vi "LP Send Cmd Done.vi"(8 "error in (no error)":errorcluster, 10 "CMD":string, 11 "Data":variant) -> ()   [LabVIEW 2015]
uses:
  Stream/Controls/RT Streamer Queue element.ctl
  Stream/Controls/RT Streamer State.ctl
  Stream/RT Controls/RT Streamer Ack element.ctl
  Stream/LP Globals.vi
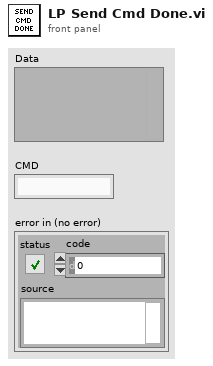
[diagram p1: front panel]
types:
  T1 = typedef "RT Streamer Ack element.ctl" = cluster{"Data":variant, "CMD":string, "error":errorcluster}
  T2 = typedef "RT Streamer Queue element.ctl" = cluster{"CMD":T3, "Data":variant}
  T3 = typedef "RT Streamer State.ctl" = enum16{"Init", "Idle", "Stream", "Listen", "SetRefrashRate", "SendCmdAck", "SendCmdDone", "SendSysState", "StartRecord", "Error"}
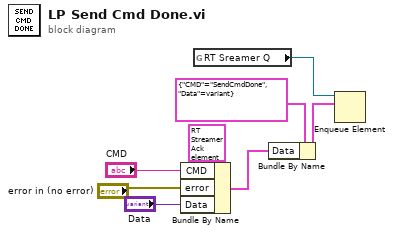
[diagram p0: block diagram]
diagram:
  n1 = Bundle By Name(cluster=T1 {"Data"=variant, "CMD"="", "error"={"status"=FALSE, "code"=0, "source"=""}} ("Cluster"), "CMD"="CMD", "error"="error in (no error)", "Data"="Data") -> (w4:T1)
  n2 = global read "LP Globals.vi" "RT Sreamer Q"() -> (w7:refnum<queue>)
  n3 = Bundle By Name(cluster=T2 {"CMD"=enum."SendCmdDone", "Data"=variant} ("element"), "Data"=w4) -> (w2:T2)
  n4 = Enqueue Element(queue=w7, element=w2) -> ()  [unwired: 2 in, 3 out]
